vi "Enable Disable Add Remove buttons.vi"(8 "error in (no error)":errorcluster, 9 "Not imported item Indexes":i32[](array[numeric]), 10 "Selected item indexes":i32[](array[numeric]), 11 "SE UI cluster in":T1={"Node Ptr"=18446744073709551615, "Add"=refnum, "Remove"=refnum, "Registers ListBox"=refnum} {"Node Ptr" format="%.0x"}) -> (0 "error out":errorcluster, 3 "SE UI cluster out":T1={"Node Ptr"=18446744073709551615, "Add"=refnum, "Remove"=refnum, "Registers ListBox"=refnum} {"Node Ptr" format="%.0x"})   [LabVIEW 2018, in "FPGA Addon System Explorer.lvlib"]
uses:
  FPGA Addon System Explorer.lvlib
  Types/SE UI Cluster.ctl
  <vilib>/NI Veristand/Custom Device API/Custom Device Item Ref.ctl
  <vilib>/NI Veristand/Custom Device API/Custom Device API.lvlib
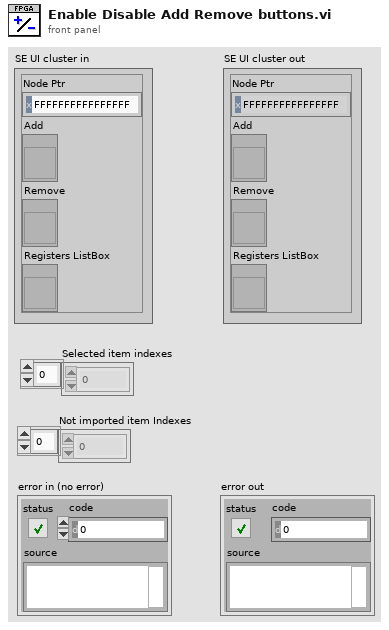
[diagram p1: front panel]
types:
  T1 = typedef "FPGA Addon System Explorer.lvlib/SE UI Cluster.ctl" = cluster{"Node Ptr":T2, "Add":refnum<vi>, "Remove":refnum<vi>, "Registers ListBox":refnum<vi>}
  T2 = typedef "Custom Device API.lvlib/Custom Device Item Ref.ctl" = u64
  T3 = enum8{"Enabled", "Disabled", "Disabled and Grayed Out"}
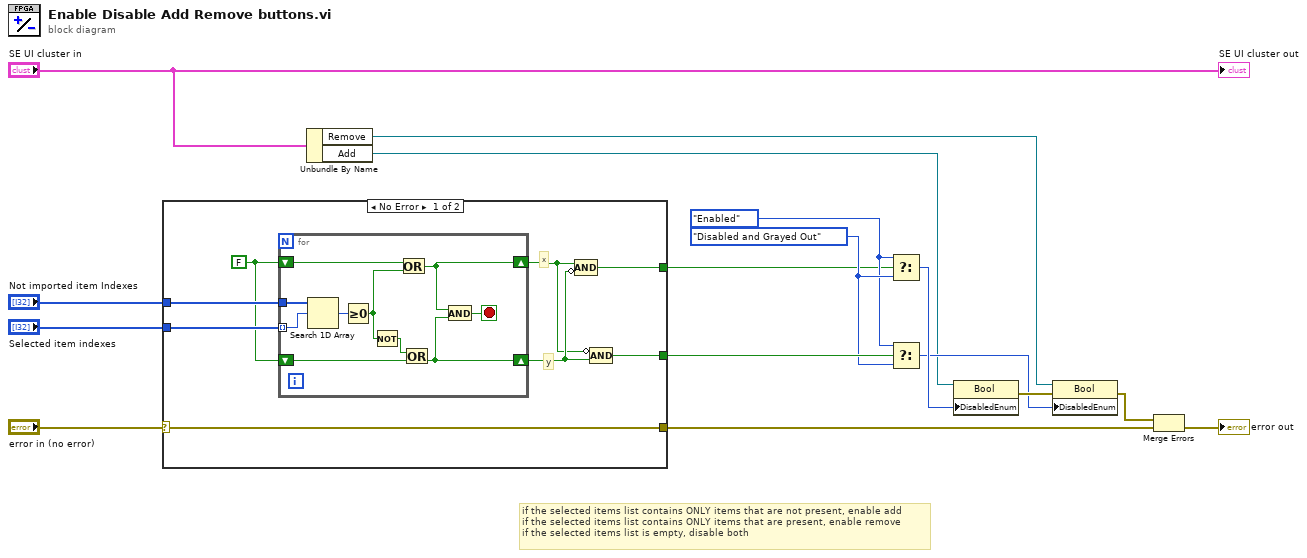
[diagram p0: block diagram]
diagram:
  w10 = T3."Disabled and Grayed Out" ("Disabled")
  w9 = T3."Enabled" ("Disabled")
  # "if the selected items list contains ONLY items that are not present, enable add\nif the selected items list contains ONLY items that are present, enable remove\nif the selected items list is empty, disable both"
  n1 = case shown="No Error" "error in (no error)" {
    selector: "error in (no error)" -> [w17 w35]
    tunnel: "Selected item indexes" -> [w24 _]
    tunnel: "Not imported item Indexes" -> [w23 _]
    tunnel: [w19 _] -> w11
    tunnel: [w18 _] -> w6
    tunnel: [w17 w35] -> w4
    frame No Error {
      w22 = FALSE
      # "y"
      # "x"
      n2 = for {
        tunnel: w24 -> [w33] mode=indexing
        tunnel: w23 -> [w34]
        shift-right: [w25] -> w20
        shift-left: w22 -> [w27]
        shift-right: [w28] -> w21
        shift-left: w22 -> [w30]
        stop <- w29 stop-if-true
        n3 = Search 1D Array(1D array=w34, element=w33) -> (index of element=w32:i32)  [unwired: 1 in]
        n4 = Greater Or Equal To 0?(x=w32) -> (x >= 0?=w26:bool)
        n5 = Not(x=w26) -> (.not. x?=w31:bool)
        n6 = Or(x=w27, y=w26) -> (x .or. y?=w25:bool)
        n7 = Or(x=w31, y=w30) -> (x .or. y?=w28:bool)
        n8 = And(x=w25, y=w28) -> (x .and. y?=w29:bool)
      }
      n9 = Compound Arithmetic op=AND(w20, invert w21) -> (w18:bool)
      n10 = Compound Arithmetic op=AND(invert w20, w21) -> (w19:bool)
    }
    frame Error {
    }
  }
  n11 = Unbundle By Name("SE UI cluster in") -> ("Remove"=w8:refnum<vi>, "Add"=w7:refnum<vi>)
  n12 = Select(t=w9, s=w6, f=w10) -> (s? t:f=w13:T3)
  n13 = Select(t=w9, s=w11, f=w10) -> (s? t:f=w12:T3)
  n14 = property on="Property Node" class="Bool"(reference=w7, "DisabledEnum"=w13) -> (error out=w15:errorcluster)  [unwired: 1 in, 1 out]
  n15 = property on="Property Node" class="Bool"(reference=w8, error in=w15, "DisabledEnum"=w12) -> (error out=w3:errorcluster)  [unwired: 1 out]
  n16 = Merge Errors(w3, w4) -> (→"error out":errorcluster)
  "SE UI cluster out" <- "SE UI cluster in"
